vi "Get Proto Value from Enum Value.vi"(8 "error in (no error)":errorcluster, 9 "enum name":string, 10 "value in LV":u32, 11 "gRPC ID in":T1) -> (0 "error out":errorcluster, 2 "value in proto":i32, 3 "gRPC ID out":T1)   [LabVIEW 2024, in "grpc-lvsupport.lvlib"]
uses:
  grpc-lvsupport.lvlib
  <resource>/grpc_labview.dll
  Shared/grpcId.ctl
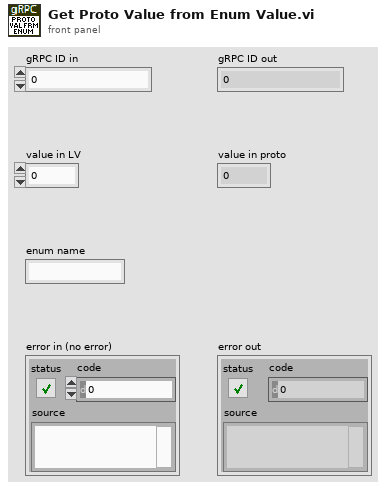
[diagram p1: front panel]
types:
  T1 = typedef "grpc-lvsupport.lvlib/grpcId.ctl" = u64
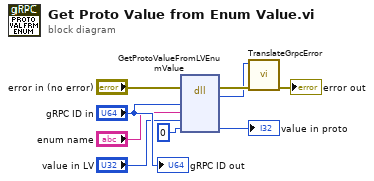
[diagram p0: block diagram]
diagram:
  n1 = dll-call lib="C:/Program Files (x86)/National Instruments/LabVIEW 2024/resource/grpc_labview.*" fn="GetProtoValueFromLVEnumValue"(error in="error in (no error)", "gRPC ID in"="gRPC ID in", "enum name"="enum name", "value in LV"="value in LV", "value in proto"=0) -> (error out=w7:errorcluster, "error code"=w6:i32, "value in proto"=→"value in proto":i32)  [unwired: 5 in, 1 out]
  n2 = call "TranslateGrpcError.vi"("error in"=w7, "Error Code"=w6) -> ("error out"=→"error out":errorcluster)  [unwired: 9 in]
  "gRPC ID out" <- "gRPC ID in"
